vi "FlatToRichcif_manager_PluginVersion.vi"(5 "OutputClusterType":T1, 11 "InputCluster":T2) -> (3 "OutputCluster":T1)   [LabVIEW 2021, in "CIF_Manager_client.lvlib"]
uses:
  CIF_Manager_client.lvlib
  cif_manager_PluginVersion_Flat.ctl
  cif_manager_PluginVersion.ctl
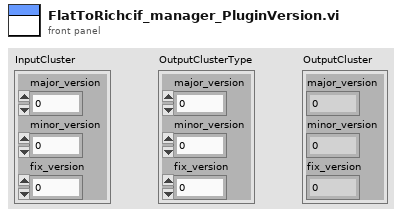
[diagram p1: front panel]
types:
  T1 = typedef "CIF_Manager_client.lvlib/cif_manager_PluginVersion.ctl" = cluster{"major_version":i32, "minor_version":i32, "fix_version":i32}
  T2 = typedef "CIF_Manager_client.lvlib/cif_manager_PluginVersion_Flat.ctl" = cluster{"major_version":i32, "minor_version":i32, "fix_version":i32}
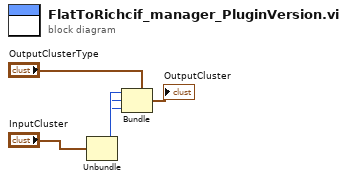
[diagram p0: block diagram]
diagram:
  n1 = Unbundle "Unbundle"("InputCluster") -> ("major_version"=w3:i32, "minor_version"=w2:i32, "fix_version"=w1:i32)
  n2 = Bundle "Bundle"(cluster="OutputClusterType", "major_version"=w3, "minor_version"=w2, "fix_version"=w1) -> (→"OutputCluster":T1)
